vi "go to return fuel.vi"(0 "system status in":T2={"system state"=enum."Empty & Closed", "fuel level"=0.0, "LOX level"=0.0, "system warnings"={"oxidizer overpress"=FALSE, "oxidizer leak"=FALSE, "fuel overpress"=FALSE, "fuel leak"=FALSE}, "valves"={"fuel load"=FALSE, "fuel return"=FALSE, "fuel comb"=FALSE, "fuel dump"=FALSE, "LOX load"=FALSE, "LOX return"=FALSE, "LOX comb"=FALSE, "LOX dump"=FALSE}, "ignition"=FALSE}, 11 "rocket controls":T1, 15 "fuel leak":bool) -> (4 "system status out":T2={"system state"=enum."Empty & Closed", "fuel level"=0.0, "LOX level"=0.0, "system warnings"={"oxidizer overpress"=FALSE, "oxidizer leak"=FALSE, "fuel overpress"=FALSE, "fuel leak"=FALSE}, "valves"={"fuel load"=FALSE, "fuel return"=FALSE, "fuel comb"=FALSE, "fuel dump"=FALSE, "LOX load"=FALSE, "LOX return"=FALSE, "LOX comb"=FALSE, "LOX dump"=FALSE}, "ignition"=FALSE})   [LabVIEW 2017]
doc: "This subVI handles the logic going to the return fuel state for the rocket engine simulation.\nIt sets the state enum to the return fuel state when the return fuel button is pushed or there is a fuel leak detected."
uses:
  typedefs/sysyem status.ctl
  typedefs/system state.ctl
  typedefs/rocket system warnings.ctl
  typedefs/user controls.ctl
panel:
  # "Standard\nProcedures"
  # "Alternate\nProcedures"
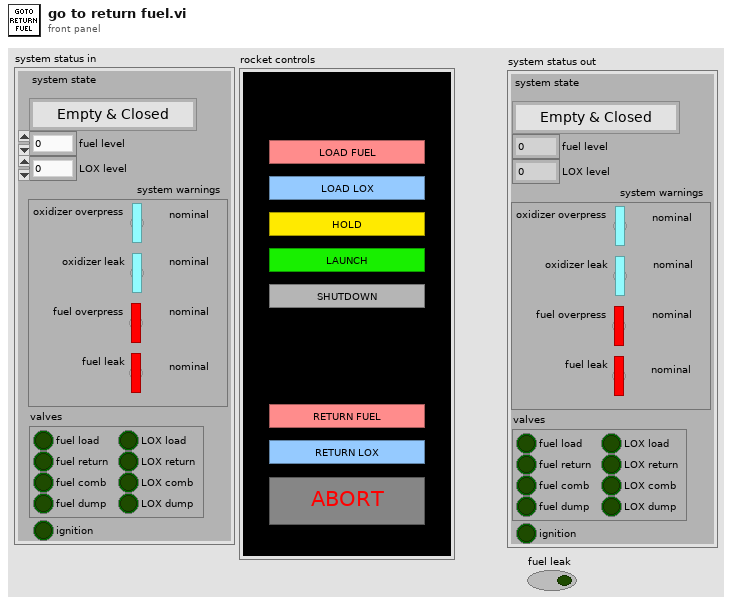
[diagram p1: front panel]
types:
  T1 = typedef "user controls.ctl" = cluster{"load fuel":bool, "load lox":bool, "hold":bool, "launch":bool, "shutdown":bool, "return fuel":bool, "return lox":bool, "abort":bool}
  T2 = typedef "sysyem status.ctl" = cluster{"system state":T3, "fuel level":dbl, "LOX level":dbl, "system warnings":T4, "valves":cluster{"fuel load":bool, "fuel return":bool, "fuel comb":bool, "fuel dump":bool, "LOX load":bool, "LOX return":bool, "LOX comb":bool, "LOX dump":bool}, "ignition":bool}
  T3 = typedef "system state.ctl" = enum16{"Hold", "Empty & Closed", "Launch", "Return Fuel", "Return LOX", "Loading Lox", "Loading Fuel", "Shutdown", "Abort"}
  T4 = typedef "rocket system warnings.ctl" = cluster{"oxidizer overpress":bool, "oxidizer leak":bool, "fuel overpress":bool, "fuel leak":bool}
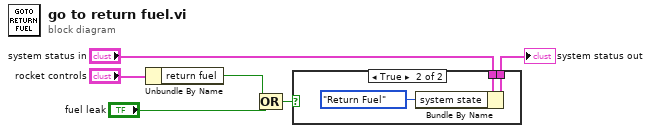
[diagram p0: block diagram]
diagram:
  n1 = Unbundle By Name("rocket controls") -> ("return fuel"=w3:bool)
  n2 = Compound Arithmetic op=OR(w3, "fuel leak") -> (w2:bool)
  n3 = case shown="True" w2 {
    tunnel: "system status in" -> [w7 w10]
    tunnel: [w7 w9] -> w5
    frame False {
    }
    frame True {
      n4 = Bundle By Name(cluster=w10, "system state"=system_state."Return Fuel") -> (w9:T2)
    }
  }
  "system status out" <- w5
